vi "DCP551DriverServer.vi"   [LabVIEW 2010, in "DCP551.lvlib"]
uses:
  DCP551.lvlib
  CM51/Comunication Status.ctl
types:
  T1 = enum32{"Invalid", "Standard", "Closed", "Hidden", "Minimized", "Maximized"}
  T2 = enum32{"invalid app kind", "Development System", "Run Time System", "Student Edition", "Embedded LabVIEW", "Evaluation", "Custom"}
  T3 = cluster{"Core":cluster{"Current VI Reference":refnum<vi>, "Close Panel on Exit?":bool}, "Serial Config":cluster{"串口选择":refnum<visa-resource-name>, "通讯速率":u32, "超时时间":u32, "数据位长":u16, "奇偶校验":enum16{"None", "Odd", "Even", "Mark", "Space"}, "停止位长":u16, "握手控制":u16, "字符结束":bool, "结束字符":u8, "仪器地址":u32}, "Your string data":string}
  T4 = cluster{"Current VI Reference":refnum<vi>, "Close Panel on Exit?":bool}
  T5 = cluster{"串口选择":refnum<visa-resource-name>, "通讯速率":u32, "超时时间":u32, "数据位长":u16, "奇偶校验":enum16{"None", "Odd", "Even", "Mark", "Space"}, "停止位长":u16, "握手控制":u16, "字符结束":bool, "结束字符":u8, "仪器地址":u32}
  T6 = cluster{"259W":string, "260W":string, "261W":string, "262W":string, "263W":string, "264W":string, "265W":string, "266W":string, "267W":string, "268W":string, "269W":string}
  T7 = cluster{"Start":enum16{"Non PV start", "Upward PV tart", "Downward PV start", "Either upward of downward PV start"}, "Cycle data":i32, "Pattern link data":i32, "Tag data":string}
  T8 = cluster{"SP":dbl, "Time":cluster{"Type":enum16{"Time Data", "delta Dtada", "SP Data"}, "Data":i32}, "EV1 to 16":cluster{"Event 1st data":i32, "Event 2nd data":i32}[], "Output limiter group data":i32, "PID group data":i32, "Repeat return segment data":i32, "Repeat data":i32, "G. soak type data":enum16{"G. soak setting is not provided", "Segment start point", "Segment end point", "Total segment"}, "G. soak width data":i32, "PV shift data":i32}[]
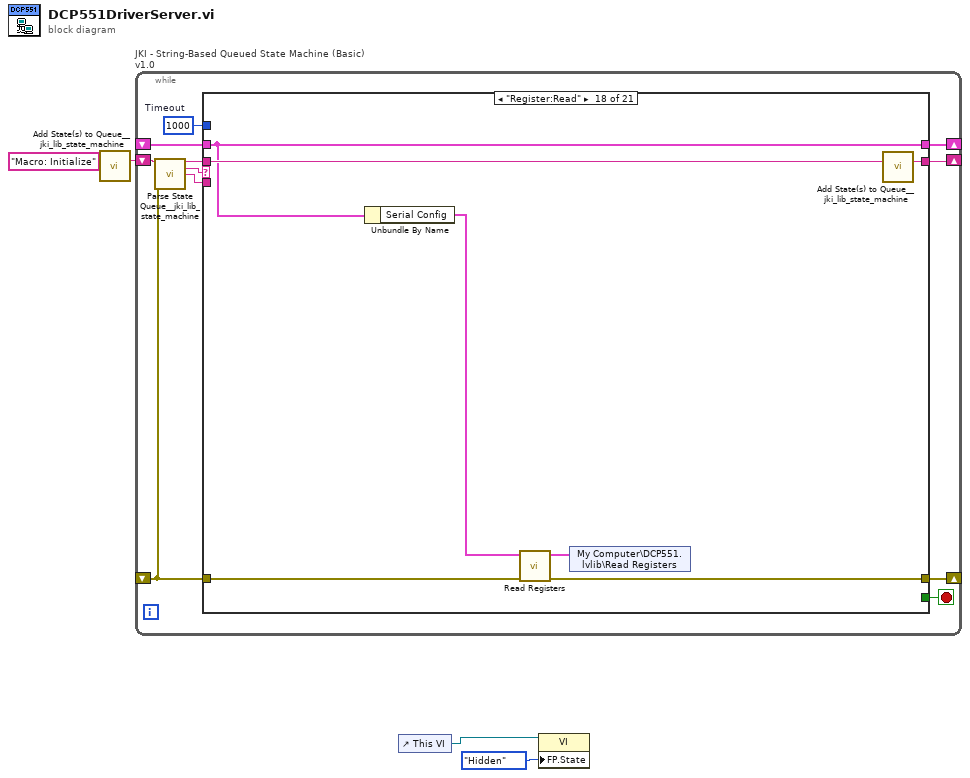
[diagram p0: block diagram]
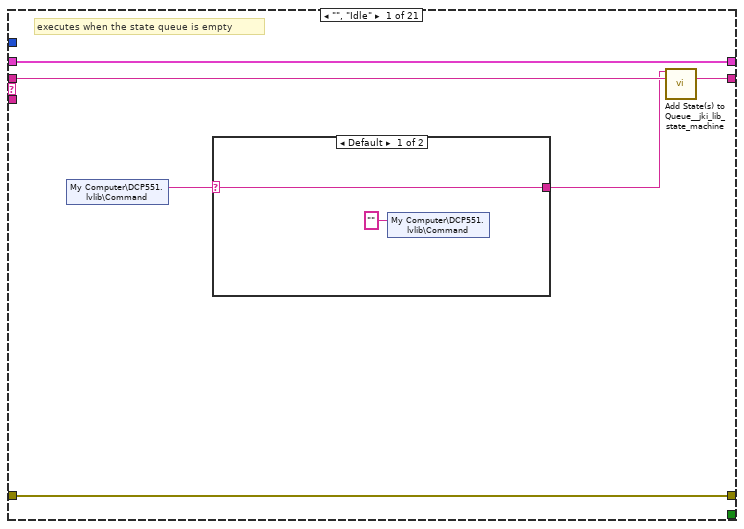
[diagram p2: hidden frame]
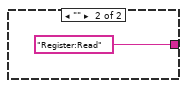
[diagram p3: hidden frame]
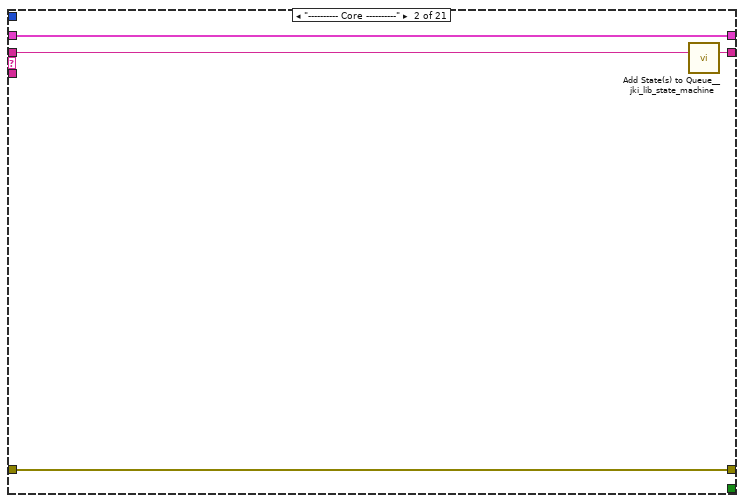
[diagram p4: hidden frame]
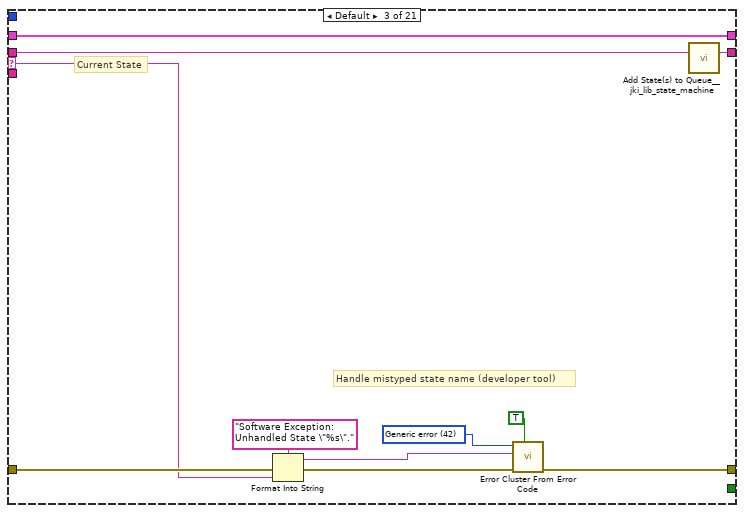
[diagram p5: hidden frame]
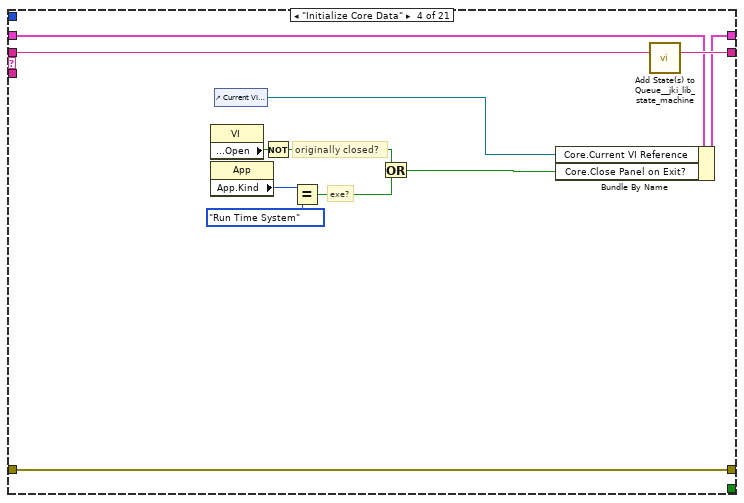
[diagram p6: hidden frame]
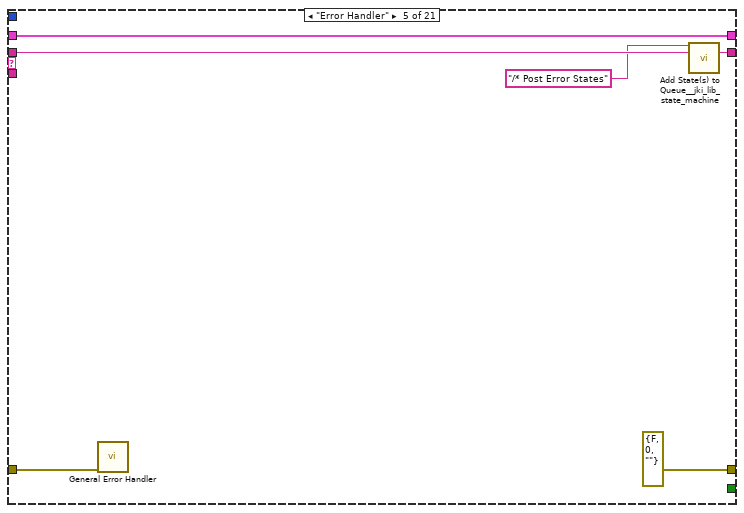
[diagram p7: hidden frame]
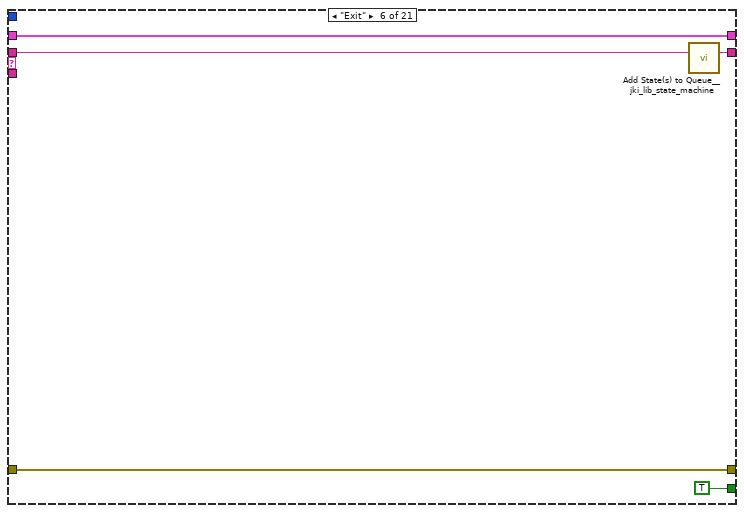
[diagram p8: hidden frame]
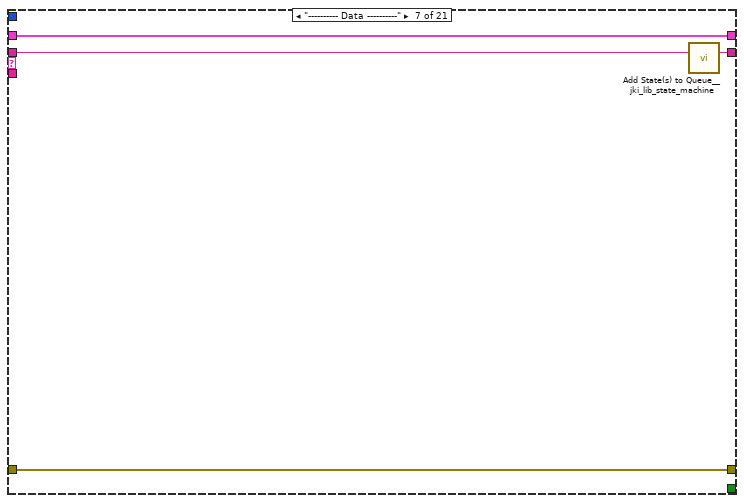
[diagram p9: hidden frame]
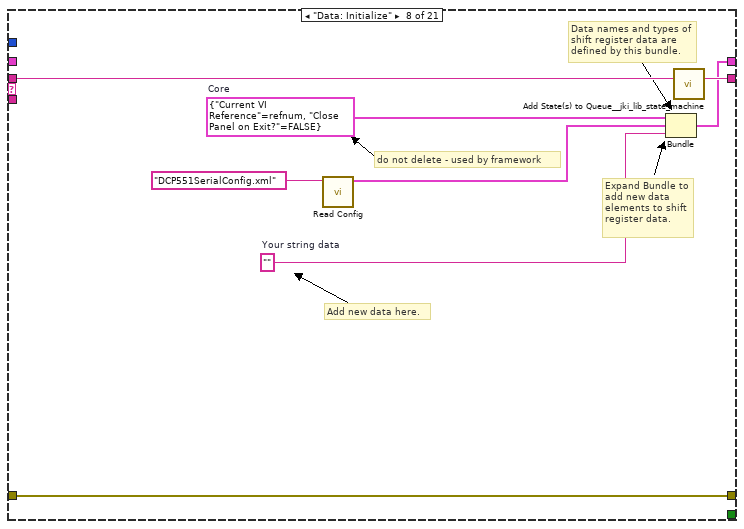
[diagram p10: hidden frame]
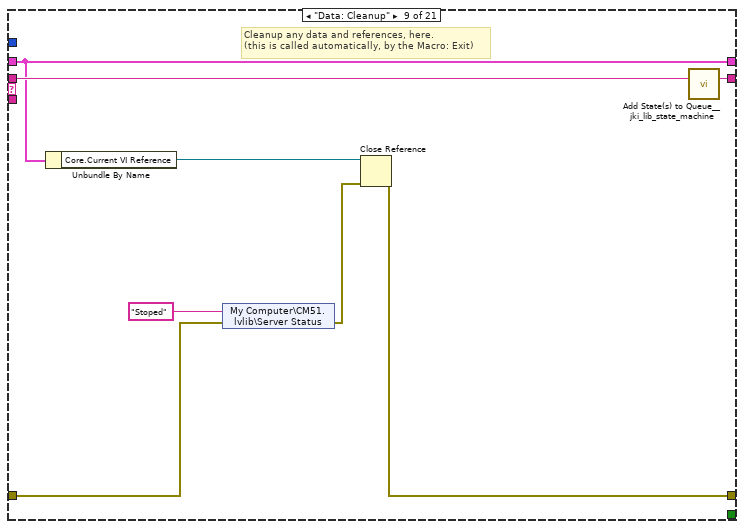
[diagram p11: hidden frame]
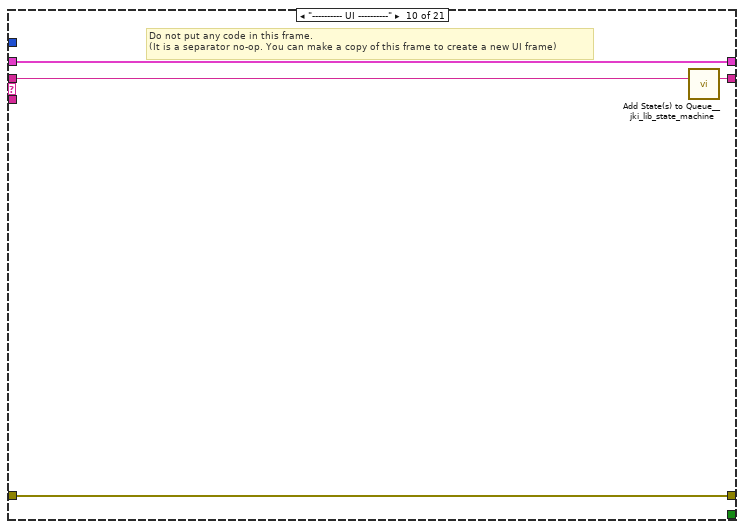
[diagram p12: hidden frame]
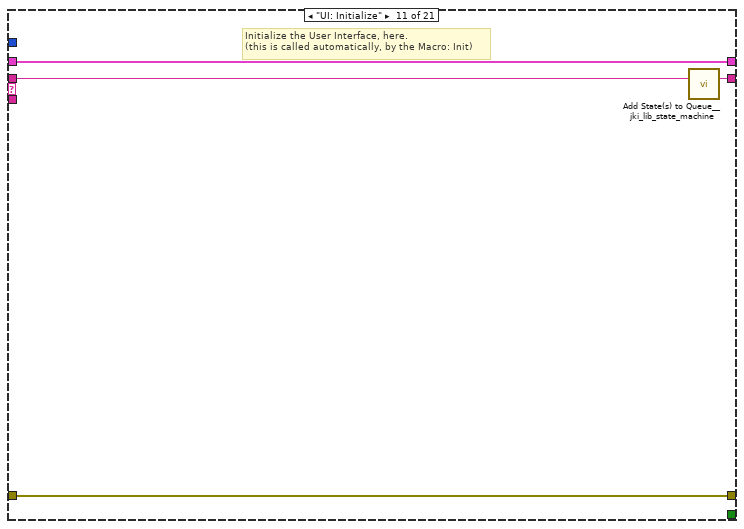
[diagram p13: hidden frame]
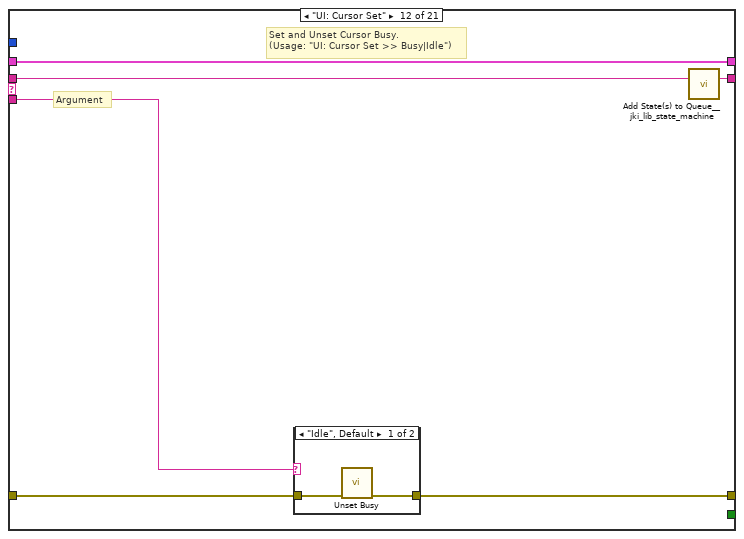
[diagram p14: hidden frame]
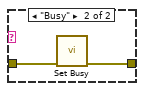
[diagram p15: hidden frame]
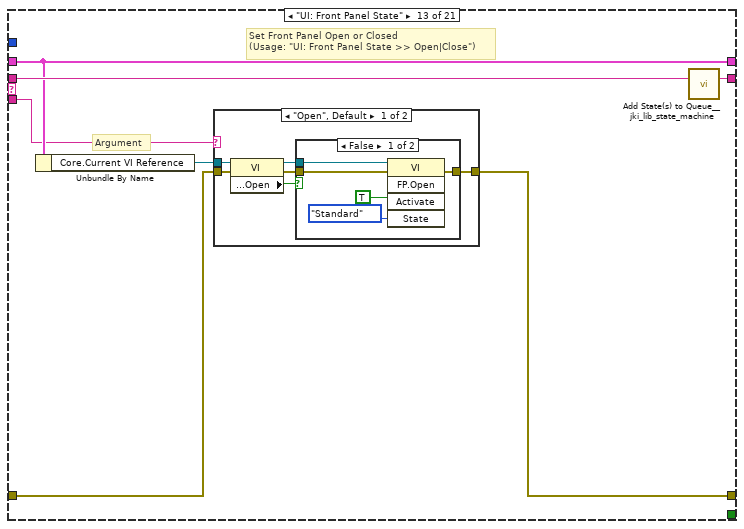
[diagram p16: hidden frame]
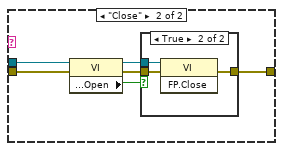
[diagram p18: hidden frame]
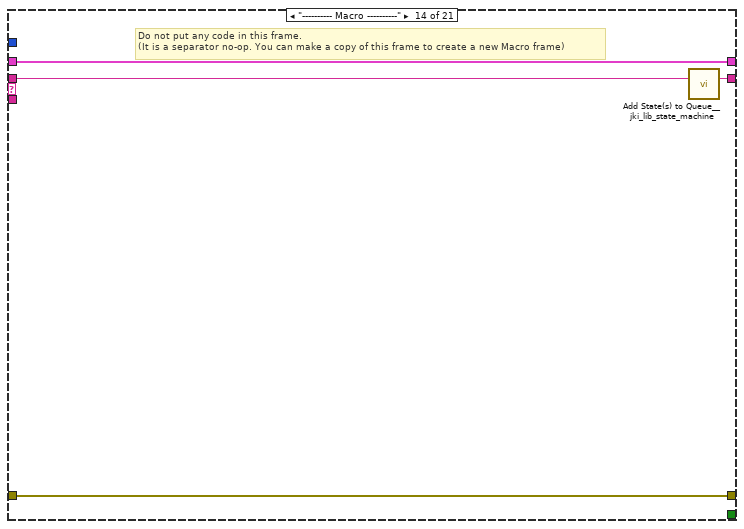
[diagram p20: hidden frame]
diagram:
  n1 = call "Add State(s) to Queue__jki_lib_state_machine.vi"("State(s) in (\"\")"="Macro: Initialize") -> ("States Out"=w4:string)  [unwired: 14 in]
  n2 = while "JKI - String-Based Queued State Machine (Basic) v1.0" {
    shift-right: [w8] -> _
    shift-left: _ -> [w7]
    shift-right: [w11] -> _
    shift-left: _ -> [w5]
    shift-right: [w10] -> _
    shift-left: w4 -> [w12]
    stop <- w9 stop-if-true
    w6 = 1000  # Timeout
    n3 = call "Parse State Queue__jki_lib_state_machine.vi"("State Queue"=w12, "Error In (no error)"=w5) -> ("Remaining States"=w14:string, "Current State"=w15:string, "Arguments"=w13:string)  [unwired: 11 in]
    n4 = case shown="\"Register:Read\"" w15 {
      selector: w15 -> [_ _ w29 _ _ _ _ _ _ _ _ _ _ _ _ _ _ _ _ _ _]
      tunnel: w14 -> [w20 w28 w33 w51 w57 w62 w66 w74 w82 w86 w90 w96 w107 w133 w138 w148 w152 w159 w165 w178 w184]
      tunnel: w13 -> [_ _ _ _ _ _ _ _ _ _ _ w91 w101 _ _ _ _ _ _ _ _]
      tunnel: w7 -> [w21 w25 w31 w42 w54 w60 w63 _ w78 w83 w88 w94 w103 w130 w135 w145 w149 w156 w161 w176 w180]
      tunnel: [w16 w26 w35 w48 errorcluster {"status"=FALSE, "code"=0, "source"=""} ("error out") w59 w64 w71 w79 w84 w87 w92 w104 w131 w136 w146 w150 w153 w162 w173 w181] -> w11
      tunnel: w5 -> [w16 w26 w34 w48 w53 w59 w64 w71 w75 w84 w87 w93 w105 w131 w136 w146 w150 w154 w163 w174 w182]
      tunnel: [w19 w27 w32 w50 w56 w61 w65 w73 w81 w85 w89 w95 w106 w132 w137 w147 w151 w158 w164 w177 w183] -> w10
      tunnel: [_ _ _ _ _ TRUE _ _ _ _ _ _ _ _ _ _ _ _ _ _ _] -> w9
      tunnel: [w21 w25 w31 w49 w54 w60 w63 w72 w78 w83 w88 w94 w103 w130 w135 w145 w149 w156 w161 w176 w180] -> w8
      tunnel: w6 -> [_ _ _ _ _ _ _ _ _ _ _ _ _ _ _ _ _ _ _ _ _]
      frame "", "Idle" {
        # "executes when the state queue is empty"
        n5 = shared-variable "My Computer\\DCP551.lvlib\\Command"() -> (w18:string)  [unwired: 1 in, 1 out]
        n6 = case shown="Default" w18 {
          selector: w18 -> [w23 _]
          tunnel: [w23 "Register:Read"] -> w17
          frame Default {
            n7 = shared-variable "My Computer\\DCP551.lvlib\\Command"("" ("Command")) -> ()  [unwired: 1 in, 1 out]
          }
          frame "" {
          }
        }
        n8 = call "Add State(s) to Queue__jki_lib_state_machine.vi"("State(s) in Front (\"\")"=w17, "State(s) in (\"\")"=w20) -> ("States Out"=w19:string)  [unwired: 13 in]
      }
      frame "---------- Core ----------" {
        n9 = call "Add State(s) to Queue__jki_lib_state_machine.vi"("State(s) in (\"\")"=w28) -> ("States Out"=w27:string)  [unwired: 14 in]
      }
      frame Default {
        w38 = 42 items=["No error", "Argument error", "Memory is full", "Out of zone", "End of file", "File already open", "Generic file I/O error", "File not found", "File permission error", "Disk is full", "Duplicate path", "Too many files open", "System feature not enabled", "Resource file not found", "Cannot add resource", "Resource not found", "Image not found", "Image memory error", "Pen does not exist", "Config type invalid", "Config token not found", "Config parse error", "Config memory error", "Bad external code format", "Bad external code offset", "External code not present", "Null window", "Destroy window error", "Null menu", "Print aborted", "Bad print record", "Print driver error", "Windows error during printing", "Memory error during printing", "Print dialog error", "Generic print error", "Invalid device refnum", "Device not found", "Device parameter error", "Device unit error", "Cannot open device", "Device call aborted", "Generic error", "Cancelled by user", "Object ID too low", "Object ID too high", "Object not in heap", "Unknown heap", "Unknown object (invalid DefProc)", "Unknown object (DefProc not in table)", "Message out of range", "Invalid (null) method", "Unknown message", "Manager call not supported", "Bad address", "Network operation in progress", "Network operation timed out", "Connection is busy", "Network attribute not supported", "Network error", "Address in use", "System out of memory", "Connection aborted", "Connection refused", "Not connected", "Already connected", "Connection closed", "Initialization error (interapplication manager)", "Bad occurrence", "Wait on unbound occurrence handler", "Occurrence queue overflow", "Datalog type conflict", "Unused", "Unrecognized type (interapplication manager)", "Memory corrupt", "Failed to make temporary DLL", "Old CIN version", "Drag socket not found", "Failed to load drop-object", "Failed to register OLE object", "Failed to release OLE object", "Format specifier type mismatch", "Unknown format specifier", "Too few format specifiers", "Too many format specifiers", "Scan failed", "Newer CIN version", "Error converting to variant", "Runtime menu error", "Password tampered", "Variant attribute not found", "Incompatible variant data type", "Event data is not available", "Event Store is not present", "Occurrence is not found", "Event Queue is not created", "Event info is not available", "Refnum passed is NULL", "Error retrieving Class GUID", "Error retrieving CoClass GUID", "Error retrieving TypeLib GUID.", "Bad built application magic bytes.", "Specific driver is different from the specific driver associated with the Logical Name.", "There is no session opened to the class driver.", "Max Error", "MAX - Error with config objects", "MAX - Error loading configuration", "MAX - Group not supported"]
        # "Current State"
        # "Handle mistyped state name (developer tool)"
        n10 = Format Into String(format string="Software Exception: Unhandled State \"%s\"." ("message"), error in=w34, w29) -> (resulting string=w37:string, error out=w36:errorcluster)  [unwired: 1 in]
        n11 = call <vilib>:"Error Cluster From Error Code.vi"("show call chain? (False)"=TRUE, "error in (no error)"=w36, "error message (\"\")"=w37, "error code (0)"=w38) -> ("error out"=w35:errorcluster)  [unwired: 5 in]
        n12 = call "Add State(s) to Queue__jki_lib_state_machine.vi"("State(s) in (\"\")"=w33) -> ("States Out"=w32:string)  [unwired: 14 in]
      }
      frame "Initialize Core Data" {
        # "originally closed?"
        # "exe?"
        n13 = property class="VI"() -> ("Front Panel.Open"=w47:bool)  [unwired: 2 in, 2 out]
        n14 = property class="App"() -> ("App.Kind"=w46:T2)  [unwired: 2 in, 2 out]
        n15 = control-ref of="Current VI Reference"() -> (w40:refnum<vi>)
        n16 = Not(x=w47) -> (.not. x?=w44:bool)
        n17 = Equal?(x=w46, y=T2."Run Time System" ("Application:Kind")) -> (x = y?=w43:bool)
        n18 = Or(x=w44, y=w43) -> (x .or. y?=w41:bool)
        n19 = Bundle By Name(cluster=w42, "Core.Current VI Reference"=w40, "Core.Close Panel on Exit?"=w41) -> (w49:T3)
        n20 = call "Add State(s) to Queue__jki_lib_state_machine.vi"("State(s) in (\"\")"=w51) -> ("States Out"=w50:string)  [unwired: 14 in]
      }
      frame "Error Handler" {
        n21 = call <vilib>:"General Error Handler.vi"("error in (no error)"=w53) -> ()  [unwired: 10 in, 5 out]
        n22 = call "Add State(s) to Queue__jki_lib_state_machine.vi"("State(s) in Front (\"\")"="/* Post Error States", "State(s) in (\"\")"=w57) -> ("States Out"=w56:string)  [unwired: 13 in]
      }
      frame "Exit" {
        n23 = call "Add State(s) to Queue__jki_lib_state_machine.vi"("State(s) in (\"\")"=w62) -> ("States Out"=w61:string)  [unwired: 14 in]
      }
      frame "---------- Data ----------" {
        n24 = call "Add State(s) to Queue__jki_lib_state_machine.vi"("State(s) in (\"\")"=w66) -> ("States Out"=w65:string)  [unwired: 14 in]
      }
      frame "Data: Initialize" {
        w69 = T4 {"Current VI Reference"=refnum, "Close Panel on Exit?"=FALSE}  # Core
        w70 = ""  # Your string data
        # "do not delete - used by framework"
        # "Expand Bundle to add new data elements to shift register data."
        # "Add new data here."
        # "Data names and types of shift register data are defined by this bundle."
        n25 = call "Read Config.vi"("FileName"="DCP551SerialConfig.xml") -> ("Serial Config"=w67:T5)  [unwired: 9 in, 1 out]
        n26 = Bundle("Core"=w69, "Serial Config"=w67, "Your string data"=w70) -> (w72:T3)  [unwired: 1 in]
        n27 = call "Add State(s) to Queue__jki_lib_state_machine.vi"("State(s) in (\"\")"=w74) -> ("States Out"=w73:string)  [unwired: 14 in]
      }
      frame "Data: Cleanup" {
        # "Cleanup any data and references, here.\n(this is called automatically, by the Macro: Exit)"
        n28 = Unbundle By Name(w78) -> ("Core.Current VI Reference"=w80:refnum<vi>)
        n29 = shared-variable "My Computer\\CM51.lvlib\\Server Status"("Stoped" ("Server Status"), error in=w75) -> (error out=w76:errorcluster)
        n30 = Close Reference(reference=w80, error in (no error)=w76) -> (error out=w79:errorcluster)
        n31 = call "Add State(s) to Queue__jki_lib_state_machine.vi"("State(s) in (\"\")"=w82) -> ("States Out"=w81:string)  [unwired: 14 in]
      }
      frame "---------- UI ----------" {
        # "Do not put any code in this frame.\n(It is a separator no-op. You can make a copy of this frame to create a new UI frame)"
        n32 = call "Add State(s) to Queue__jki_lib_state_machine.vi"("State(s) in (\"\")"=w86) -> ("States Out"=w85:string)  [unwired: 14 in]
      }
      frame "UI: Initialize" {
        # "Initialize the User Interface, here.\n(this is called automatically, by the Macro: Init)"
        n33 = call "Add State(s) to Queue__jki_lib_state_machine.vi"("State(s) in (\"\")"=w90) -> ("States Out"=w89:string)  [unwired: 14 in]
      }
      frame "UI: Cursor Set" {
        # "Argument"
        # "Set and Unset Cursor Busy.\n(Usage: \"UI: Cursor Set >> Busy|Idle\")"
        n34 = case shown="\"Idle\", Default" w91 {
          tunnel: w93 -> [w98 w100]
          tunnel: [w97 w99] -> w92
          frame "Idle", Default {
            n35 = call <vilib>:"Unset Busy.vi"("error in (no error)"=w98) -> ("error out"=w97:errorcluster)  [unwired: 10 in]
          }
          frame "Busy" {
            n36 = call <vilib>:"Set Busy.vi"("error in (no error)"=w100) -> ("error out"=w99:errorcluster)  [unwired: 9 in, 1 out]
          }
        }
        n37 = call "Add State(s) to Queue__jki_lib_state_machine.vi"("State(s) in (\"\")"=w96) -> ("States Out"=w95:string)  [unwired: 14 in]
      }
      frame "UI: Front Panel State" {
        # "Argument"
        # "Set Front Panel Open or Closed\n(Usage: \"UI: Front Panel State >> Open|Close\")"
        n38 = Unbundle By Name(w103) -> ("Core.Current VI Reference"=w102:refnum<vi>)
        n39 = case shown="\"Open\", Default" w101 {
          tunnel: w105 -> [w111 w124]
          tunnel: [w113 w125] -> w104
          tunnel: w102 -> [w112 w122]
          frame "Open", Default {
            n40 = property class="VI"(reference=w112, error in=w111) -> (reference out=w109:refnum<vi>, error out=w110:errorcluster, "Front Panel.Open"=w108:bool)
            n41 = case shown="False" w108 {
              tunnel: [w116 w119] -> w113
              tunnel: w110 -> [w115 w119]
              tunnel: w109 -> [w114 _]
              frame False {
                n42 = invoke class="VI" method="FP.Open"(reference=w114, error in=w115, "Activate"=TRUE, "State"=T1."Standard") -> (error out=w116:errorcluster)  [unwired: 1 in, 4 out]
              }
              frame True {
              }
            }
          }
          frame "Close" {
            n43 = property class="VI"(reference=w122, error in=w124) -> (reference out=w121:refnum<vi>, error out=w123:errorcluster, "Front Panel.Open"=w120:bool)
            n44 = case shown="True" w120 {
              tunnel: [w126 w129] -> w125
              tunnel: w123 -> [w126 w128]
              tunnel: w121 -> [_ w127]
              frame False {
              }
              frame True {
                n45 = invoke class="VI" method="FP.Close"(reference=w127, error in=w128) -> (error out=w129:errorcluster)  [unwired: 1 in, 2 out]
              }
            }
          }
        }
        n46 = call "Add State(s) to Queue__jki_lib_state_machine.vi"("State(s) in (\"\")"=w107) -> ("States Out"=w106:string)  [unwired: 14 in]
      }
      frame "---------- Macro ----------" {
        # "Do not put any code in this frame.\n(It is a separator no-op. You can make a copy of this frame to create a new Macro frame)"
        n47 = call "Add State(s) to Queue__jki_lib_state_machine.vi"("State(s) in (\"\")"=w133) -> ("States Out"=w132:string)  [unwired: 14 in]
      }
      frame "Macro: Initialize" {
        w134 = "Data: Initialize\nInitialize Core Data\nUI: Initialize\nUI: Front Panel State >> Open"  # Data: Initialize Initialize Core Data UI: Initialize UI: Front Panel State >> Open
        # "Initialization Macro\n(This is called once, when the VI starts)"
        n48 = call "Add State(s) to Queue__jki_lib_state_machine.vi"("State(s) in Front (\"\")"=w134, "State(s) in (\"\")"=w138) -> ("States Out"=w137:string)  [unwired: 13 in]
      }
      frame "Macro: Exit" {
        # "Exit Macro\n(This is called once, when the VI exits)"
        n49 = Unbundle By Name(w145) -> ("Core.Close Panel on Exit?"=w144:bool)
        n50 = Select(t="UI: Front Panel State >> Close", s=w144, f="") -> (s? t:f=w141:string)
        n51 = call "Add State(s) to Queue__jki_lib_state_machine.vi"("State(s) in (\"\")"=w141, "State(s) at Back (\"\")"="Data: Cleanup\nExit") -> ("States Out"=w139:string)  [unwired: 13 in]
        n52 = call "Add State(s) to Queue__jki_lib_state_machine.vi"("State(s) in Front (\"\")"=w139, "State(s) in (\"\")"=w148) -> ("States Out"=w147:string)  [unwired: 13 in]
      }
      frame "---------- New Category ----------" {
        # "Template Separator\n(You can make a copy of, or modify, this frame)"
        n53 = call "Add State(s) to Queue__jki_lib_state_machine.vi"("State(s) in (\"\")"=w152) -> ("States Out"=w151:string)  [unwired: 14 in]
      }
      frame "Register:Read" {
        n54 = Unbundle By Name(w156) -> ("Serial Config"=w157:T5)
        n55 = call "Read Registers.vi"("error in (no error)"=w154, "Serial Config"=w157) -> ("error out"=w153:errorcluster, "Registers"=w155:T6)  [unwired: 7 in, 1 out]
        n56 = shared-variable "My Computer\\DCP551.lvlib\\Read Registers"(w155) -> ()  [unwired: 1 in, 1 out]
        n57 = call "Add State(s) to Queue__jki_lib_state_machine.vi"("State(s) in (\"\")"=w159) -> ("States Out"=w158:string)  [unwired: 14 in]
      }
      frame "Register:Write" {
        n58 = Unbundle By Name(w161) -> ("Serial Config"=w160:T5)
        n59 = call "Write Registers.vi"("error in (no error)"=w163, "Serial Config"=w160) -> ("error out"=w162:errorcluster)  [unwired: 8 in, 1 out]
        n60 = call "Add State(s) to Queue__jki_lib_state_machine.vi"("State(s) in (\"\")"=w165) -> ("States Out"=w164:string)  [unwired: 14 in]
      }
      frame "File:Read" {
        n61 = Unbundle By Name(w176) -> ("Serial Config"=w175:T5)
        n62 = shared-variable "My Computer\\DCP551.lvlib\\File ID"() -> (w172:string)  [unwired: 1 in, 1 out]
        n63 = call "Read File.vi"("File ID"=w172, "error in (no error)"=w174, "Serial Config"=w175) -> ("error out"=w173:errorcluster, "Segment 0"=w171:T7, "Segment 1 to 99"=w170:T8)  [unwired: 6 in]
        n64 = shared-variable "My Computer\\DCP551.lvlib\\Segment 1 to 99"(w170) -> (error out=w168:errorcluster)  [unwired: 1 in]
        n65 = shared-variable "My Computer\\DCP551.lvlib\\Segment0"(w171) -> (error out=w167:errorcluster)  [unwired: 1 in]
        n66 = Merge Errors(w168, w167) -> (w166:errorcluster)
        n67 = shared-variable "My Computer\\DCP551.lvlib\\Server Status"("Read Over" ("Server Status"), error in=w166) -> ()  [unwired: 1 out]
        n68 = call "Add State(s) to Queue__jki_lib_state_machine.vi"("State(s) in (\"\")"=w178) -> ("States Out"=w177:string)  [unwired: 14 in]
      }
      frame "File:Write" {
        n69 = flat-sequence {
          tunnel: w182 -> [w191]
          tunnel: w180 -> [w189]
          tunnel: [w190] -> w179
          tunnel: [w193] -> w181
          tunnel: w179 -> [w193]
          frame #0 {
            n70 = shared-variable "My Computer\\DCP551.lvlib\\File ID"() -> (w185:string)  [unwired: 1 in, 1 out]
            n71 = shared-variable "My Computer\\DCP551.lvlib\\Segment0"() -> (w186:T7)  [unwired: 1 in, 1 out]
            n72 = shared-variable "My Computer\\DCP551.lvlib\\Segment 1 to 99"() -> (w187:T8)  [unwired: 1 in, 1 out]
            n73 = Unbundle By Name(w189) -> ("Serial Config"=w188:T5)
            n74 = call "Write File.vi"("File ID"=w185, "error in (no error)"=w191, "Segment 1 to 99"=w187, "Segment 0"=w186, "Serial Config"=w188) -> ("error out"=w190:errorcluster)  [unwired: 6 in]
          }
          frame #1 {
            n75 = shared-variable "My Computer\\DCP551.lvlib\\Server Status"("Working" ("Server Status")) -> ()  [unwired: 1 in, 1 out]
          }
        }
        n76 = call "Add State(s) to Queue__jki_lib_state_machine.vi"("State(s) in (\"\")"=w184) -> ("States Out"=w183:string)  [unwired: 14 in]
      }
    }
  }
  n77 = control-ref of="This VI"() -> (w2:refnum<vi>)
  n78 = property class="VI"(reference=w2, "FP.State"=T1."Hidden" ("Front Panel Window:State")) -> ()  [unwired: 1 in, 2 out]
